vi "Modbus MicroZed.vi"(8 "Error In":errorcluster, 9 "port (502)":u16=502, 10 "address":string, 11 "PC Config":T3={"AC Voltage SP"=0.0, "AC Current SP"=0.0, "Frequency SP"=60.0, "DC Voltage SP"=0.0, "Op Mode SP"=enum."Shutdown (Reset)", "Clear Faults SP"=0} {"Clear Faults SP" format="%01x"; "DC Voltage SP" min=300 max=550 format="%2.1f"; "Frequency SP" min=45 max=65 format="%2.1f"; "AC Current SP" min=-500 max=500 format="%2.1f"; "AC Voltage SP" min=0 max=132 format="%2.1f"}) -> (0 "Error Out":errorcluster, 3 "PC Data":T1 {"Alarms 2" format="%016b"; "Faults 2" format="%016b"; "Alarms 1" format="%016b"; "Faults 1" format="%016b"; "Contactor FB" format="%.0b"; "DC Voltage SP" format="%2.1f"; "Clear Faults SP" format="%.0b"; "Neutral Current" format="%2.1f"; "AC Current - L2" format="%2.1f"; "AC Voltage - L2" format="%2.1f"; "Temperature" format="%2.1f"; "DC Voltage" format="%2.1f"; "AC Current SP" format="%2.1f"; "AC Voltage SP" format="%2.1f"; "Frequency SP" format="%2.1f"; "AC Frequency" format="%2.1f"; "AC Current - L1" format="%2.1f"; "AC Voltage- L1" format="%2.1f"})   [LabVIEW 2014]
uses:
  Controls/ModbusState.ctl
  <vilib>/Modbus/master/Modbus Master.lvclass
  Controls/MicroZed Config.ctl
  Controls/MicroZed Config Op Mode.ctl
  Controls/PC Data.ctl
  <vilib>/Modbus/master/Create Master Instance (TCP).vi
panel:
  out "TCP Master Ref Out":refnum<class "Modbus Master.lvclass">
  out "Modbus State Out":T4
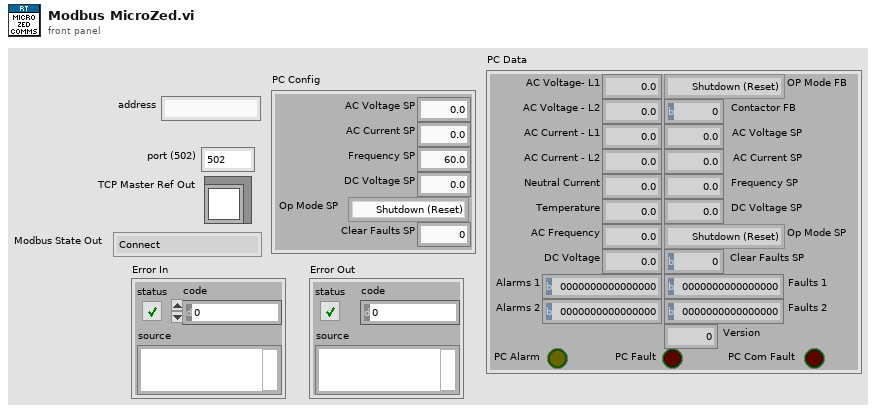
[diagram p1: front panel]
types:
  T1 = typedef "PC Data.ctl" = cluster{"AC Voltage- L1":dbl, "AC Voltage - L2":dbl, "AC Current - L1":dbl, "AC Current - L2":dbl, "Neutral Current":dbl, "Temperature":dbl, "AC Frequency":dbl, "DC Voltage":dbl, "AC Voltage SP":dbl, "AC Current SP":dbl, "Frequency SP":dbl, "Op Mode SP":T2, "Clear Faults SP":u16, "PC Com Fault":bool, "PC Fault":bool, "DC Voltage SP":dbl, "OP Mode FB":T2, "Contactor FB":u16, "Faults 1":u16, "Alarms 1":u16, "Faults 2":u16, "Alarms 2":u16, "PC Alarm":bool, "Version":u16}
  T2 = typedef "MicroZed Config Op Mode.ctl" = enum16{"Shutdown (Reset)", "Startup", "Idle", "Voltage Mode", "Current Mode", "Fault", "OL Voltage (Debug)", "No Data"}
  T3 = typedef "MicroZed Config.ctl" = cluster{"AC Voltage SP":sgl, "AC Current SP":sgl, "Frequency SP":sgl, "DC Voltage SP":sgl, "Op Mode SP":T2, "Clear Faults SP":i16}
  T4 = typedef "ModbusState.ctl" = enum16{"Connect", "Disconnect", "Set Basic Objects", "Get Basic Objects", "Read", "Write", "Read/Write"}
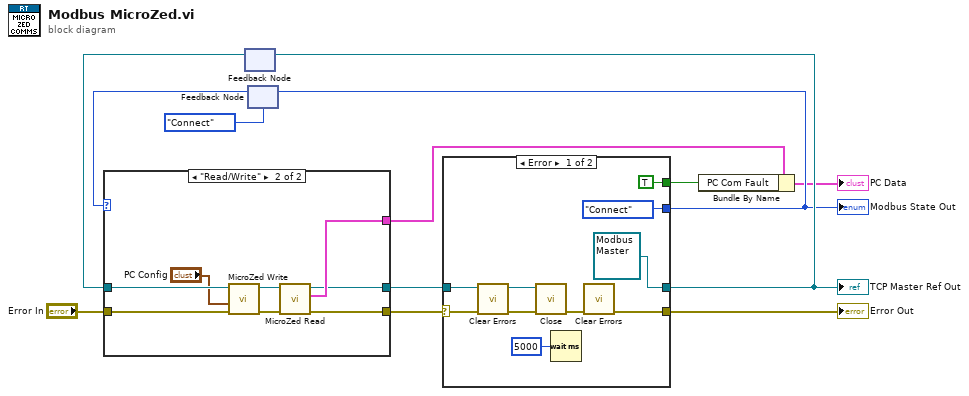
[diagram p0: block diagram]
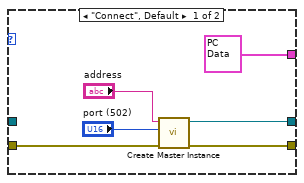
[diagram p2: hidden frame]
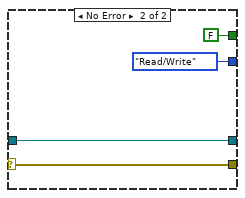
[diagram p3: hidden frame]
diagram:
  n1 = feedback #1() -> (w9:refnum<class "Modbus Master.lvclass">)  [unwired: 1 in]
  n2 = feedback #2(ModbusState."Connect" ("Modbus State In")) -> (w11:T4)
  n3 = case shown="\"Read/Write\"" w11 {
    tunnel: "Error In" -> [w18 w25]
    tunnel: [w14 w19] -> w6
    tunnel: w9 -> [_ w26]
    tunnel: [w13 w20] -> w8
    tunnel: [T1 {"AC Voltage- L1"=0.0, "AC Voltage - L2"=0.0, "AC Current - L1"=0.0, "AC Current - L2"=0.0, "Neutral Current"=0.0, "Temperature"=0.0, "AC Frequency"=0.0, "DC Voltage"=0.0, "AC Voltage SP"=0.0, "AC Current SP"=0.0, "Frequency SP"=0.0, "Op Mode SP"=enum."Shutdown (Reset)", "Clear Faults SP"=0, "PC Com Fault"=FALSE, "PC Fault"=FALSE, "DC Voltage SP"=0.0, "OP Mode FB"=enum."Shutdown (Reset)", "Contactor FB"=0, "Faults 1"=0, "Alarms 1"=0, "Faults 2"=0, "Alarms 2"=0, "PC Alarm"=FALSE, "Version"=0} ("PC Data") w21] -> w3
    frame "Connect", Default {
      n4 = call-poly <vilib>:"Create Master Instance.vi"("error in (no error)"=w18, "port (502)"="port (502)", "address"="address") -> ("error out"=w13:errorcluster, "TCP master instance"=w14:refnum<class "Modbus Master.lvclass">)  [unwired: 7 in]
    }
    frame "Read/Write" {
      n5 = call "MicroZed Write.vi"("Error In"=w25, "PC Config"="PC Config", "TCP Master Ref In"=w26) -> ("Error Out"=w24:errorcluster, "TCP Master Ref Out"=w23:refnum<class "Modbus Master.lvclass">)  [unwired: 7 in]
      n6 = call "MicroZed Read.vi"("Error In"=w24, "TCP Master Ref In"=w23) -> ("Error Out"=w20:errorcluster, "PC Data"=w21:T1, "TCP Master Ref Out"=w19:refnum<class "Modbus Master.lvclass">)  [unwired: 7 in]
    }
  }
  n7 = case shown="Error" w8 {
    selector: w8 -> [w28 w39]
    tunnel: w6 -> [w33 w38]
    tunnel: [w34 w39] -> w7
    tunnel: [refnum<class "Modbus Master.lvclass"> refnum ("TCP master instance") w38] -> w5
    tunnel: [ModbusState."Connect" ("Modbus State In") ModbusState."Read/Write" ("Modbus State In")] -> w4
    tunnel: [TRUE FALSE] -> w2
    frame Error {
      n8 = call <vilib>:"Clear Errors.vi"("error in (no error)"=w28) -> ("error out"=w29:errorcluster)  [unwired: 5 in, 1 out]
      n9 = call-dynamic "Close.vi"("error in (no error)"=w29, "Modbus master in"=w33) -> ("error out"=w35:errorcluster)  [unwired: 9 in]
      n10 = Wait (ms)(milliseconds to wait=u32 5000) -> ()  [unwired: 1 out]
      n11 = call <vilib>:"Clear Errors.vi"("error in (no error)"=w35) -> ("error out"=w34:errorcluster)  [unwired: 5 in, 1 out]
    }
    frame No Error {
    }
  }
  "Error Out" <- w7
  "Modbus State Out" <- w4
  "TCP Master Ref Out" <- w5
  n12 = feedback-in #1(w5) -> ()
  n13 = feedback-in #2(w4) -> ()
  n14 = Bundle By Name(cluster=w3, "PC Com Fault"=w2) -> (→"PC Data":T1)
